vi "Listen.vi"(8 "error in (no error)":errorcluster, 9 "Timeout":i32, 11 "Execution Profiler In":refnum<class "Execution Profiler.lvclass">) -> (0 "error out":errorcluster, 3 "Execution Profiler Out":refnum<class "Execution Profiler.lvclass">)   [LabVIEW 2020, in "Execution Profiler.lvclass"]
uses:
  Execution Profiler.lvclass
  Execution Profiler View.vi
  Execution Profiler Result View/Execution Profiler Result View.lvclass
  Execution Profiler View Data.ctl
  Helper Classes/Open Test Case Interface/Open Test Case.lvclass
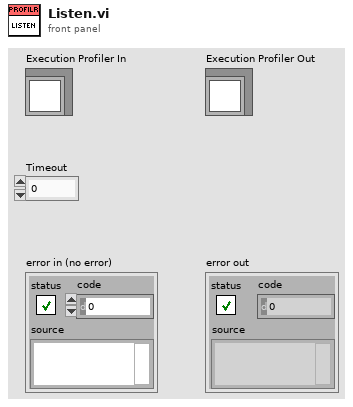
[diagram p1: front panel]
types:
  T1 = typedef "Execution Profiler Result View.lvclass/Execution Profiler View Data.ctl" = cluster{"Timing Results":map{string, dbl}, "Tags":string[], "Test Finder":refnum<class "Open Test Case.lvclass">}
  T2 = typedef "Test Case Result.lvlib/Test Case Result type.ctl" = map{string, T3}
  T3 = typedef "Method Result.lvlib/Method Result type.ctl" = cluster{"Test Case":string, "Test Method Name":string, "Status":T4, "Assertion Results":T5[], "Execution time":dbl, "Result String":string}
  T4 = typedef "Assertion Result.lvlib/Status.ctl" = enum16{"Pass", "Fail", "Error", "Skipped", "Setup Error", "Broken", "Teardown Error"}
  T5 = typedef "Assertion Result.lvlib/Assertion Result type.ctl" = cluster{"Status":T4, "Message":string, "Description":string, "Assertion Type":T6}
  T6 = typedef "Assertion Result.lvlib/Assertion Type.ctl" = enum16{"None", "Pass", "Fail", "Skip", "Pass if Equal", "Fail if Equal", "Pass if Error", "Fail if Error", "Pass if", "Fail if"}
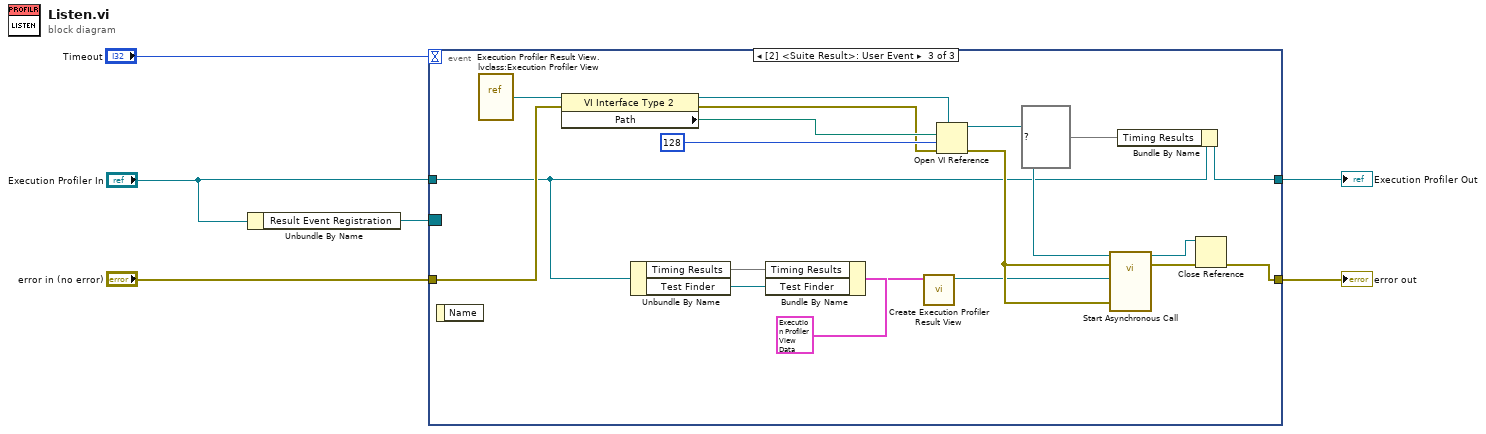
[diagram p0: block diagram]
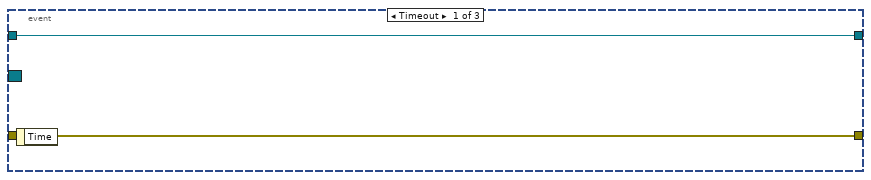
[diagram p2: hidden frame]
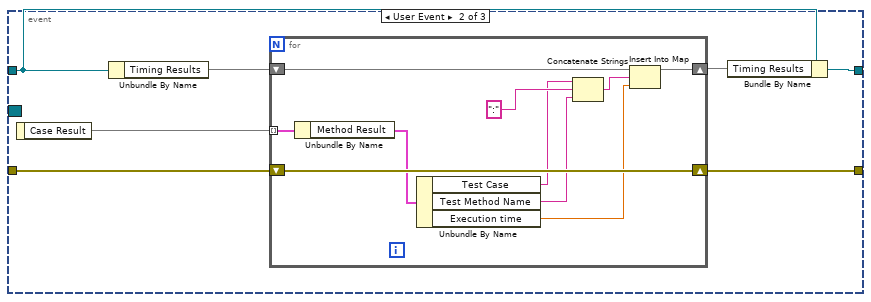
[diagram p3: hidden frame]
diagram:
  n1 = Unbundle By Name("Execution Profiler In") -> ("Result Event Registration"=w3:refnum<event-registration>)
  n2 = event shown="[2] <Suite Result>: User Event" {
    selector: w3 -> [_ _ _]
    dyn-events: _ -> [_ _ _]
    timeout: "Timeout" -> [_ _ _]
    tunnel: "error in (no error)" -> [w8 w10 w34]
    tunnel: [w8 w15 w35] -> w4
    tunnel: "Execution Profiler In" -> [w7 w13 w30]
    tunnel: [w7 w11 w33] -> w1
    event Timeout {
      n3 = event-data() -> ()  [unwired: 1 in, 1 out]
    }
    event User Event {
      n4 = event-data() -> ("Case Result"=w9:T2)  [unwired: 1 in]
      n5 = Unbundle By Name(w13) -> ("Timing Results"=w14:map{string, dbl})
      n6 = for {
        tunnel: w9 -> [w21] mode=indexing
        shift-right: [w20] -> w15
        shift-left: w10 -> [w20]
        shift-right: [w22] -> w12
        shift-left: w14 -> [w23]
        n7 = Unbundle By Name(w21) -> ("Method Result"=w19:T3)
        n8 = Unbundle By Name(w19) -> ("Test Case"=w18:string, "Test Method Name"=w17:string, "Execution time"=w16:dbl)
        n9 = Concatenate Strings(w18, ":" ("string"), w17) -> (w24:string)
        n10 = Insert Into Map(map in=w23, key=w24, value=w16) -> (map out=w22:map{string, dbl})  [unwired: 2 out]
      }
      n11 = Bundle By Name(cluster=w13, "Timing Results"=w12) -> (w11:refnum<class "Execution Profiler.lvclass">)
    }
    event User Event {
      n12 = event-data() -> ()  [unwired: 1 in, 1 out]
      n13 = vi-ref "Execution Profiler Result View.lvclass:Execution Profiler View.vi"() -> (w37:refnum<vi>)
      n14 = property class="VI Interface Type 2"(reference=w37, error in=w34) -> (reference out=w41:refnum<vi>, error out=w39:errorcluster, "Path"=w40:path)
      n15 = Unbundle By Name(w30) -> ("Timing Results"=w29:map{string, dbl}, "Test Finder"=w28:refnum<class "Open Test Case.lvclass">)
      n16 = Bundle By Name(cluster=T1 {"Timing Results"={}, "Tags"=[], "Test Finder"=refnum} ("Data"), "Timing Results"=w29, "Test Finder"=w28) -> (w27:T1)
      n17 = call "Create Execution Profiler Result View.vi"("Execution Profiler Result View in"=w27) -> ("Execution Profiler Result View out"=w26:refnum<class "Execution Profiler Result View.lvclass">)  [unwired: 9 in, 1 out]
      n18 = Open VI Reference(type specifier VI Refnum (for type only)=w41, vi path=w40, options=128, error in (no error)=w39) -> (vi reference=w36:refnum<vi>, error out=w38:errorcluster)  [unwired: 2 in]
      n19 = call-by-ref "Start Asynchronous Call"(reference=w36, error in=w38, 8:"error in (no error)"=w38, "Execution Profiler Result View.lvclass"=w26) -> (reference out=w44:refnum<vi>, error out=w43:errorcluster)  [unwired: 9 in, 1 out]
      n20 = Bundle By Name(cluster=w30, "Timing Results"=map{string, dbl} {}) -> (w33:refnum<class "Execution Profiler.lvclass">)
      n21 = Close Reference(reference=w44, error in (no error)=w43) -> (error out=w35:errorcluster)
    }
  }
  "error out" <- w4
  "Execution Profiler Out" <- w1
